vi "Save2Excel.vi"(0 "File Path":path, 1 "File name (wo extension)":string, 2 "Type of curve to save":u16(ring)=2 items=["Save the transmission spectrum", "Save the source spectrum"], 3 "XY Graph":cluster{dbl[], "Processed Spectrum":dbl[]}, 4 "Array":cluster{dbl[], dbl[]}[](array[cluster]), 5 "error in (no error)":errorcluster) -> (19 "error out":errorcluster)   [LabVIEW 2023]
uses:
  <vilib>/Utility/file.llb/Write Delimited Spreadsheet (DBL).vi
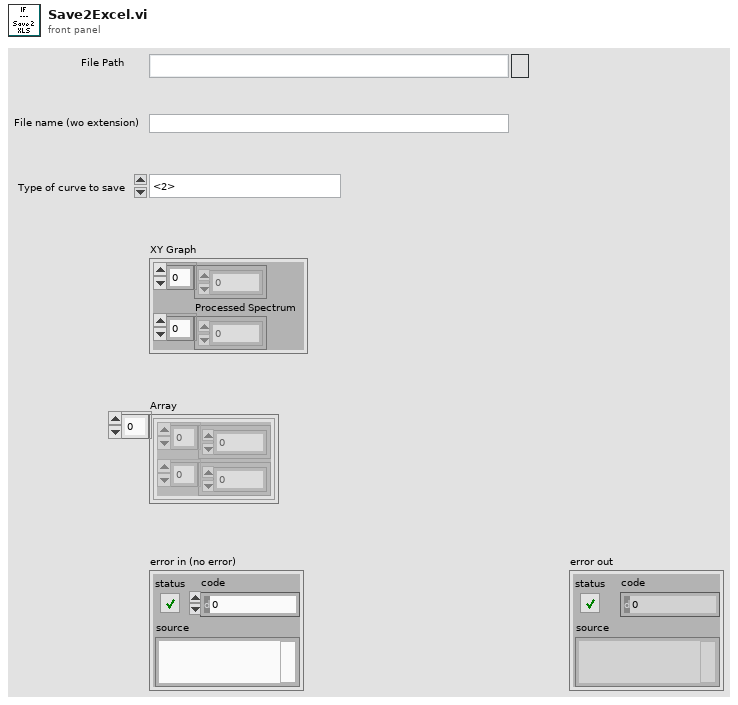
[diagram p1: front panel]
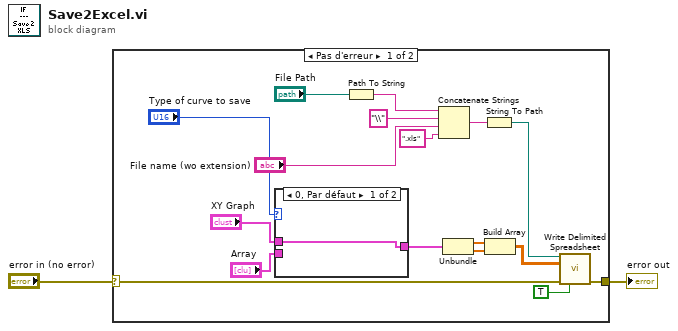
[diagram p0: block diagram]
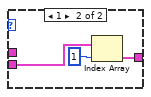
[diagram p2: hidden frame]
diagram:
  n1 = case shown="Pas d'erreur" "error in (no error)" {
    selector: "error in (no error)" -> [w3 w24]
    tunnel: [w4 w24] -> w2
    frame No Error {
      n2 = case shown="0, Par défaut" "Type of curve to save" {
        tunnel: "XY Graph" -> [w20 _]
        tunnel: "Array" -> [_ w23]
        tunnel: [w20 w21] -> w17
        frame 0, Default {
        }
        frame 1 {
          n3 = Index Array(array=w23, index=1) -> (element=w21:cluster{dbl[], dbl[]})
        }
      }
      n4 = Path To String(path="File Path") -> (string=w6:string)
      n5 = Concatenate Strings(w6, "\\", "File name (wo extension)", ".xls" ("string")) -> (w9:string)
      n6 = Unbundle(w17) -> (w18:dbl[], "Processed Spectrum"=w16:dbl[])
      n7 = String To Path(string=w9) -> (path=w10:path)
      n8 = Build Array(w18, w16) -> (w19:dbl[][])
      n9 = call-poly <vilib>:"Write Delimited Spreadsheet.vi"("file path (dialog if empty)"=w10, "2D data"=w19, "error in (no error)"=w3, "transpose? (no:F)"=TRUE) -> ("error out"=w4:errorcluster)  [unwired: 10 in, 1 out]
    }
    frame Error {
    }
  }
  "error out" <- w2
